vi "Write Events.vi"(8 "error in (no error)":errorcluster, 10 "Events":refnum<class "Event_Polled Type.lvclass">[](array[class]), 11 "Event_Source in":refnum<class "Event_Source.lvclass">) -> (0 "error out":errorcluster, 3 "Event_Source out":refnum<class "Event_Source.lvclass">)   [LabVIEW 2021, in "Event_Source.lvclass"]
uses:
  Event_Source.lvclass
  Event_Polled Type.lvclass
  C:/TSA/Omni-Bus/Source/Event Bus/Support/Event Type/Event_Type.lvclass
  Event_Source.lvclass/Event_Source.ctl
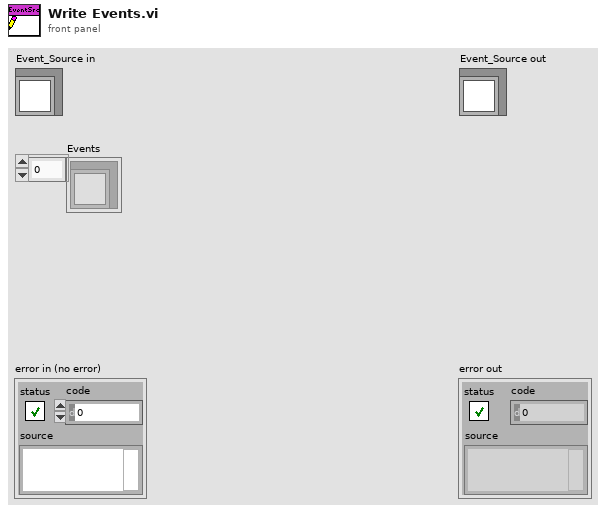
[diagram p1: front panel]
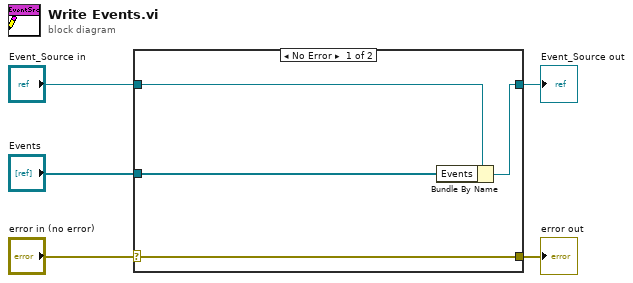
[diagram p0: block diagram]
diagram:
  n1 = case shown="No Error" "error in (no error)" {
    selector: "error in (no error)" -> [w9 w10]
    tunnel: [w9 w10] -> w4
    tunnel: [w7 w11] -> w2
    tunnel: "Event_Source in" -> [w8 w11]
    tunnel: "Events" -> [w6 _]
    frame No Error {
      n2 = Bundle By Name(cluster=w8, "Events"=w6) -> (w7:refnum<class "Event_Source.lvclass">)
    }
    frame Error {
    }
  }
  "error out" <- w4
  "Event_Source out" <- w2
